vi "TopVIPath.vi"() -> (0 "ConfigFile path":path, 1 "ResultsData path":path, 2 "LV Source":path)   [LabVIEW 2021, in "TopPath.lvlib"]
doc: "解析开发环境和Exe环境下的顶层路径。二者是不同的。20131104\n\nContact\njiangsong@outlook.com\n\n修改记录。\n修改：FilePath的路径为固定的Source里面。使用各自的文件夹。用来保存各种配置文件（只要是文件都保存在这个目录的对应子目录下），读写文件。固定于“[Project]\\Source”\nData：用来保存测试数据。 固定于“[Project]\\Data”\n2015-10-31 11:06:51\n蒋松"
uses:
  <userlib>/John_Lib/TopPath/TopPath.lvlib
  <userlib>/John_Lib/TopPath/Top Path.ctl
panel:
  out "EXE":bool
  out "TopPath":T1
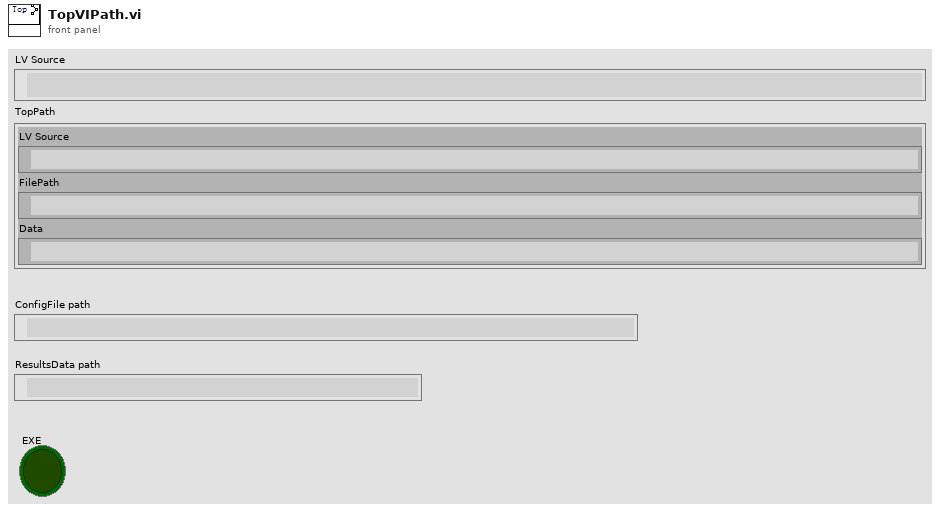
[diagram p1: front panel]
types:
  T1 = typedef "TopPath.lvlib/Top Path.ctl" = cluster{"LV Source":path, "FilePath":path, "Data":path}
  T2 = enum32{"invalid app kind", "Development System", "Run Time System", "Student Edition", "Embedded LabVIEW", "Evaluation", "Custom"}
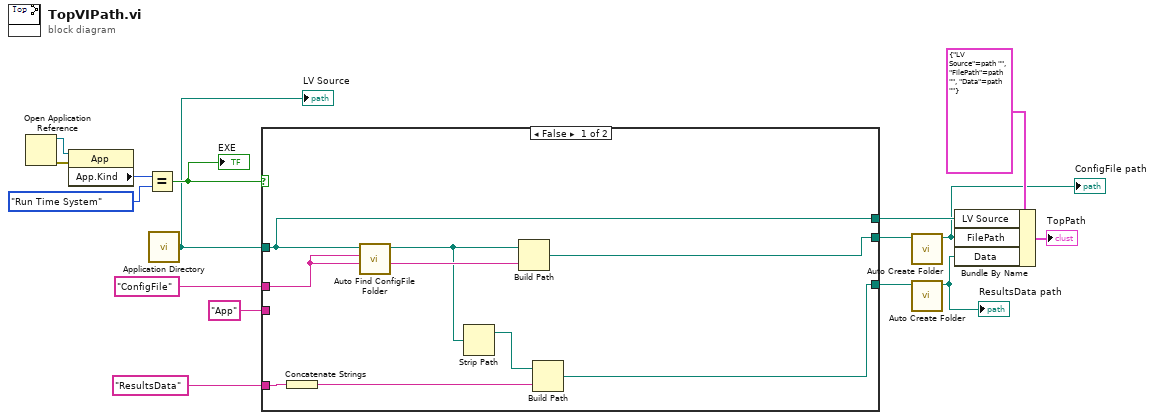
[diagram p0: block diagram]
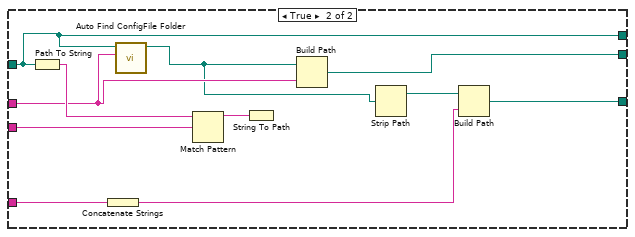
[diagram p2: hidden frame]
diagram:
  n1 = Open Application Reference() -> (0:w4:errorcluster, 3:w5:refnum<vi>)  [unwired: 4 in]
  n2 = property class="App"(reference=w5, error in=w4) -> ("App.Kind"=w3:T2)  [unwired: 2 out]
  n3 = Equal?(x=w3, y=T2."Run Time System") -> (x = y?=w16:bool)
  "EXE" <- w16
  n4 = call <vilib>:"Application Directory.vi"() -> ("Application Directory"=w15:path)
  "LV Source" <- w15
  n5 = case shown="False" w16 {
    tunnel: w15 -> [w19 w25]
    tunnel: [w19 w25] -> w13
    tunnel: [w22 w34] -> w7
    tunnel: [w21 w35] -> w9
    tunnel: "ConfigFile" ("name or relative path") -> [w18 w27]
    tunnel: "ResultsData" ("name or relative path") -> [w23 w32]
    tunnel: "App" ("regular expression") -> [_ w28]
    frame False {
      n6 = Concatenate Strings(w23) -> (w24:string)
      n7 = call <userlib>:"Auto Find ConfigFile Folder.vi"("ConfigFile"=w18, "Application Directory"=w19) -> ("Project Folder"=w17:path)  [unwired: 9 in]
      n8 = Strip Path(path=w17) -> (stripped path=w20:path)  [unwired: 1 out]
      n9 = Build Path ("[Project]\\File")(base path=w17, name or relative path=w18) -> (appended path=w21:path)
      n10 = Build Path ("[Project]外")(base path=w20, name or relative path=w24) -> (appended path=w22:path)
    }
    frame True {
      n11 = Path To String(path=w25) -> (string=w30:string)
      n12 = Concatenate Strings(w32) -> (w33:string)
      n13 = call <userlib>:"Auto Find ConfigFile Folder.vi"("ConfigFile"=w27, "Application Directory"=w25) -> ("Project Folder"=w26:path)  [unwired: 9 in]
      n14 = Match Pattern(string=w30, regular expression=w28) -> (before substring=w29:string)  [unwired: 1 in, 3 out]
      n15 = String To Path(string=w29) -> ()  [unwired: 1 out]
      n16 = Build Path(base path=w26, name or relative path=w27) -> (appended path=w35:path)
      n17 = Strip Path(path=w26) -> (stripped path=w31:path)  [unwired: 1 out]
      n18 = Build Path(base path=w31, name or relative path=w33) -> (appended path=w34:path)
    }
  }
  n19 = call <userlib>:"Auto Create Folder.vi"("Folder path"=w9) -> ("Folder path"=w8:path)  [unwired: 9 in, 1 out]
  "ConfigFile path" <- w8
  n20 = call <userlib>:"Auto Create Folder.vi"("Folder path"=w7) -> ("Folder path"=w6:path)  [unwired: 9 in, 1 out]
  "ResultsData path" <- w6
  n21 = Bundle By Name(cluster=T1 {"LV Source"=path "", "FilePath"=path "", "Data"=path ""}, "LV Source"=w13, "FilePath"=w8, "Data"=w6) -> (→"TopPath":T1)
